vi "Read_DI.vi"(8 "error in (no error)":errorcluster caption="错误输入（无错误）", 11 "Name":string[](array[string])) -> (0 "DI":bool[](array[boolean]), 3 "error":bool)   [LabVIEW 2017]
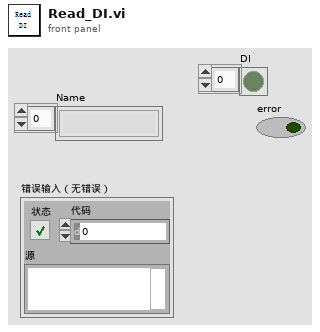
[diagram p1: front panel]
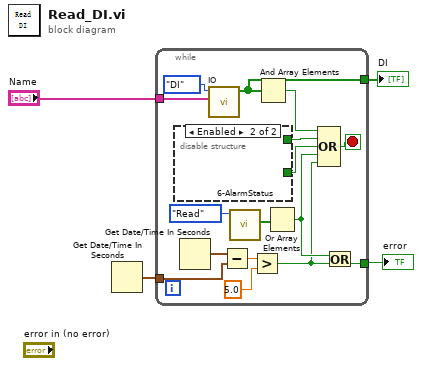
[diagram p0: block diagram]
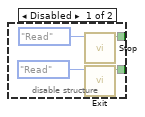
[diagram p2: hidden frame]
diagram:
  n1 = Get Date/Time In Seconds() -> (seconds since 1Jan1904=w2:timestamp)
  n2 = while {
    tunnel: "Name" -> [w16]
    tunnel: w2 -> [w12]
    tunnel: [w7] -> w4
    tunnel: [w8] -> w1
    stop <- w17 stop-if-true
    n3 = disable-structure shown="Enabled" {
      disable-tunnel: [w22 _] -> w19
      disable-tunnel: [w21 _] -> w18
      frame Disabled {
        n4 = call "Stop.vi"("Step"=enum16{"Initial", "Write", "Read"}."Read") -> ("Stop Out"=w21:bool)  [unwired: 9 in, 1 out]
        n5 = call "Exit.vi"("Step"=enum16{"Initial", "Write", "Read"}."Read" ("step")) -> ("Exit Out"=w22:bool)  [unwired: 9 in, 1 out]
      }
      frame Enabled {
      }
    }
    n6 = Get Date/Time In Seconds() -> (seconds since 1Jan1904=w13:timestamp)
    n7 = call "IO.vi"("IO Name"=w16, "IO?"=enum16{"DI", "DO"}."DI") -> ("DI"=w8:bool[])  [unwired: 7 in, 2 out]
    n8 = Subtract(x=w13, y=w12) -> (x-y=w14:dbl)
    n9 = call "6-AlarmStatus.vi"("Step"=enum16{"Initial", "Write", "Read"}."Read") -> ("AlarmValue Out"=w9:bool[])  [unwired: 9 in, 1 out]
    n10 = Greater?(x=w14, y=5.0) -> (0:w5:bool)
    n11 = And Array Elements(Boolean array=w8) -> (logical AND=w15:bool)
    n12 = Or Array Elements(Boolean array=w9) -> (logical OR=w6:bool)
    n13 = Compound Arithmetic op=OR ("复合运算")(w15, w18, w19, w6, w5) -> (w17:bool)
    n14 = Or(x=w6, y=w5) -> (x .or. y?=w7:bool)
  }
  "error" <- w4
  "DI" <- w1
